vi "Compose Cluster - String - Element Value.vi"() -> ()   [LabVIEW 2017, in "Composition.Tests.lvlib"]
uses:
  Composition.Tests.lvlib
  270ad85e-0f6a-4071-ac1f-40b2bf285315.vi
  <vilib>/addons/_JKI Toolkits/Caraya/classes/Test/Test.lvclass
  <vilib>/addons/_JKI Toolkits/Caraya/classes/Assert/Assert.lvclass
panel:
  out "error out":errorcluster
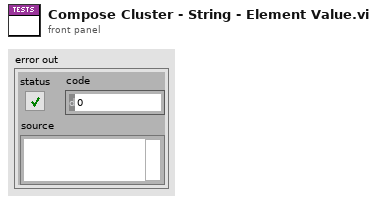
[diagram p1: front panel]
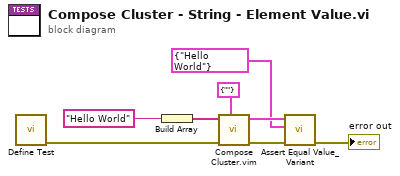
[diagram p0: block diagram]
diagram:
  n1 = call <vilib>:"Define Test.vi"() -> ("error out"=w3:errorcluster)  [unwired: 11 in]
  n2 = Build Array("Hello World") -> (w6:string[])
  n3 = call "Compose Cluster.vim"("Type"=cluster{string} {""}, "error in"=w3, "Elements"=w6) -> ("error out"=w5:errorcluster, "Cluster"=w2:cluster{string})  [unwired: 7 in]
  n4 = call <vilib>:"Assert Equal Value_Variant.vi"("error in (no error)"=w5, "Y"=cluster{string} {"Hello World"}, "X"=w2) -> ("error out"=→"error out":errorcluster)  [unwired: 8 in]
